vi "Assemble module.vi"() -> ()   [LabVIEW 2016]
uses:
  Classes/Assembly/Assembly Run.lvclass
  Classes/Routine/Routine Enum.ctl
  Classes/Workspace/Fixture Enum.ctl
  Classes/Routine/Routine.lvclass
  Classes/Workspace/Fixture.lvclass
  Classes/Controller/Controller.lvclass
panel:
  out "Routine Status":string
  in  "Add to Assembly":bool
  out "?":bool
  out "?":bool
  out "?":bool
  out "?":bool
  out "Theta":dbl
  out "Z":dbl
  out "Y":dbl
  out "X":dbl
  in  "Baseplate Tray ID":i32
  in  "Component Tray ID":i32
  out "Baseplate tray vacuum":bool
  out "Component Tray Vacuum":bool
  out "O-ring vacuum":bool
  out "Assembly vacuum":bool
  out "Component vacuum":bool
  out "Secondary vacuum":bool
  out "Primary vacuum":bool
  in  "Stop":bool
  in  "Number of modules":i32
  in  "Glue step":enum16{"Kapton", "Sensor", "PCB"}(ring)
  in  "Go":bool
  # "Status"
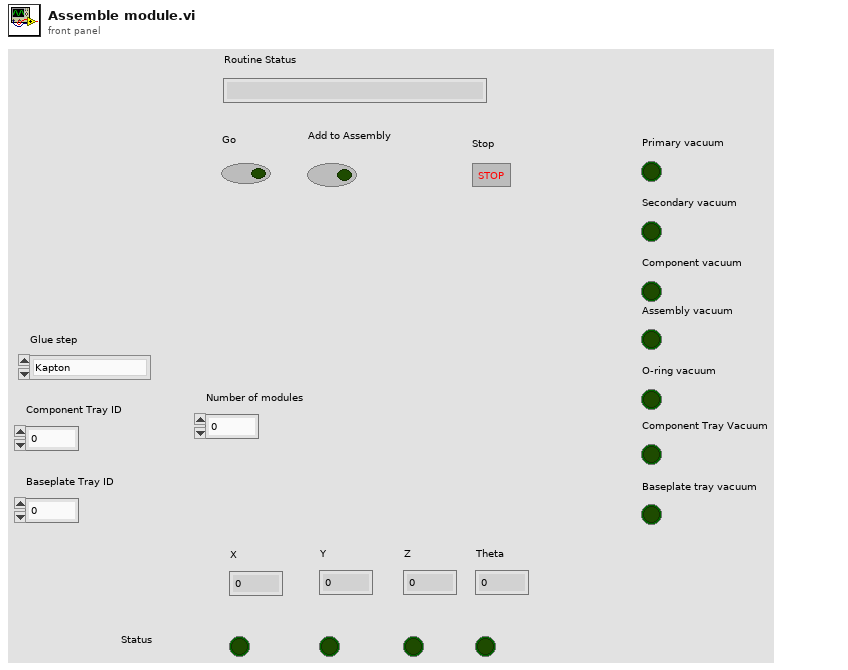
[diagram p1: front panel]
types:
  T1 = typedef "Fixture.lvclass/Fixture Enum.ctl" = enum16{"Assembly Tray", "Syringe Space", "Component", "Pick Up Tool", "Current Position"}
  T2 = typedef "Routine.lvclass/Routine Enum.ctl" = enum16{"Primary Pick Up", "Pick Up All", "Put Down Secondary", "Put Down All", "Release Syringe", "Secondary Pick Up", "Secure Syringe", "Dispense on Plate", "Dispense on Kapton", "Dispense on Sensor"}
  T3 = typedef "Controller.lvclass/Controllers.ctl" = cluster{"I-O.lvclass":refnum<class "I-O.lvclass">, "Motion.lvclass":refnum<class "Motion.lvclass">, "Dispenser.lvclass":refnum<class "Dispenser.lvclass">}
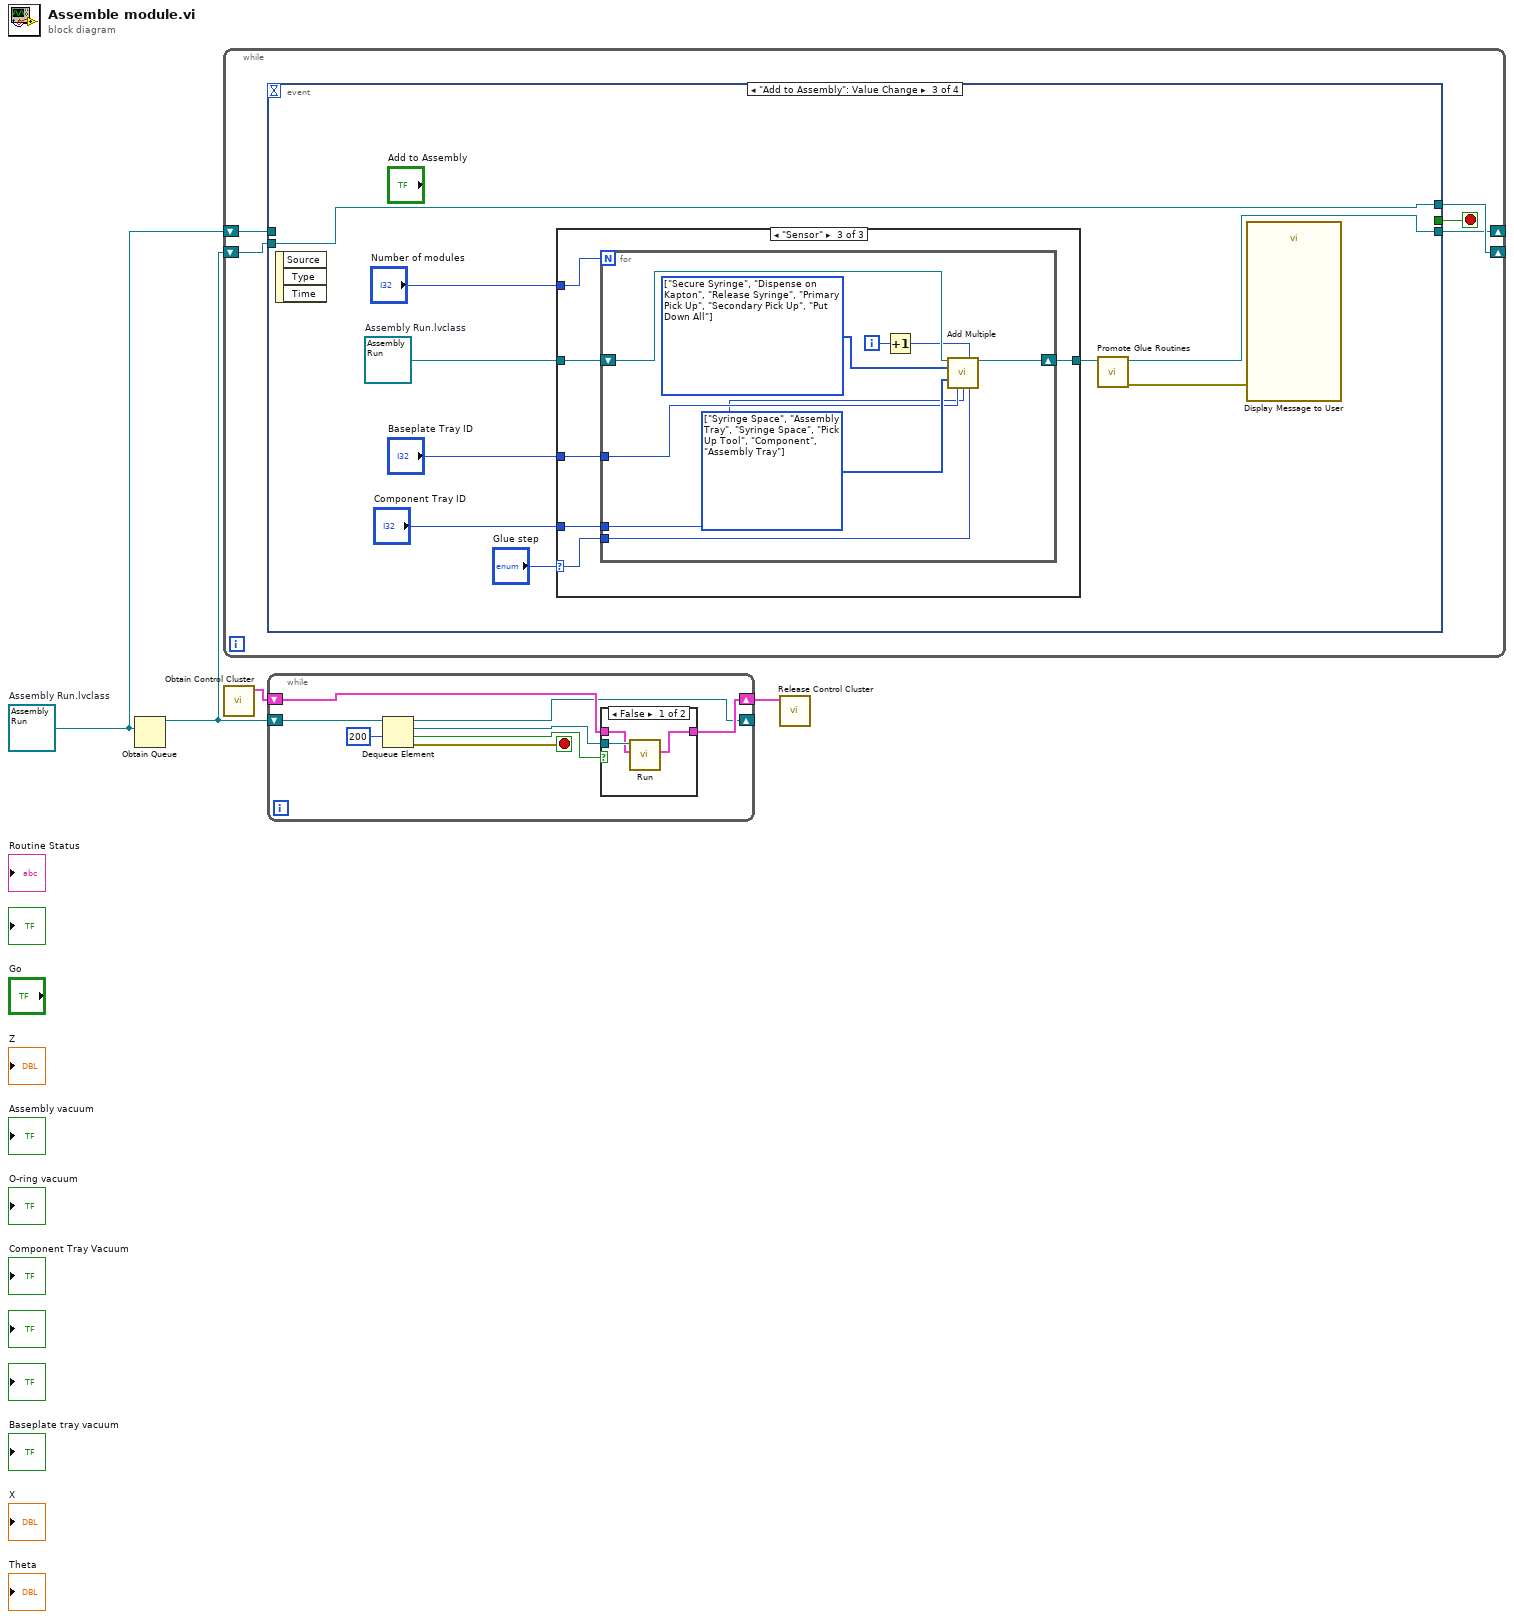
[diagram p0: block diagram]
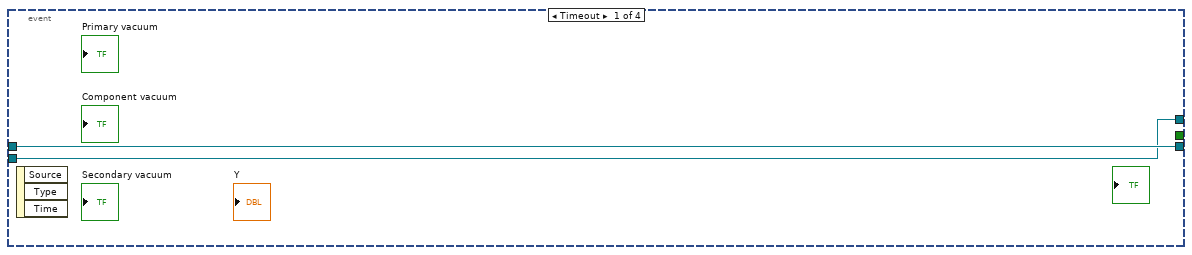
[diagram p3: hidden frame]
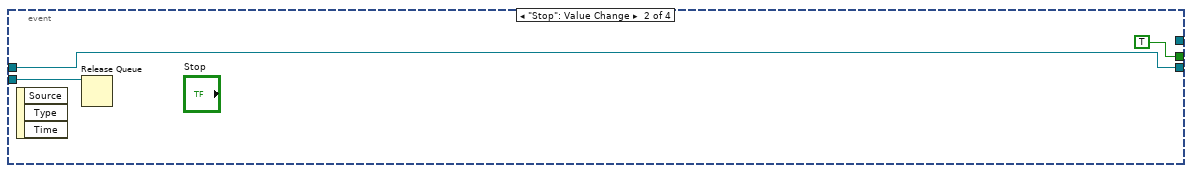
[diagram p4: hidden frame]
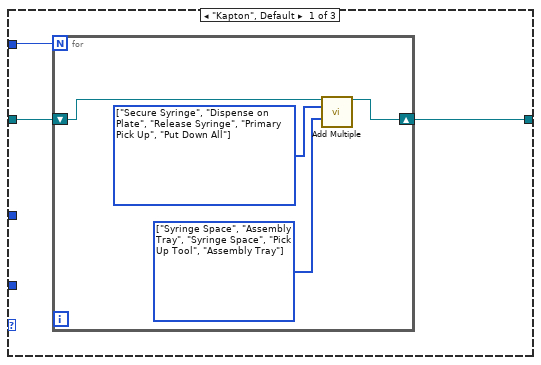
[diagram p5: hidden frame]
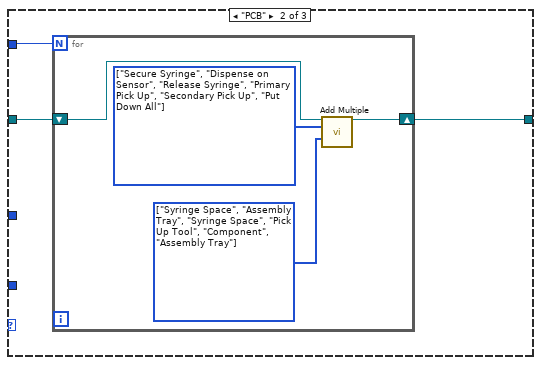
[diagram p6: hidden frame]
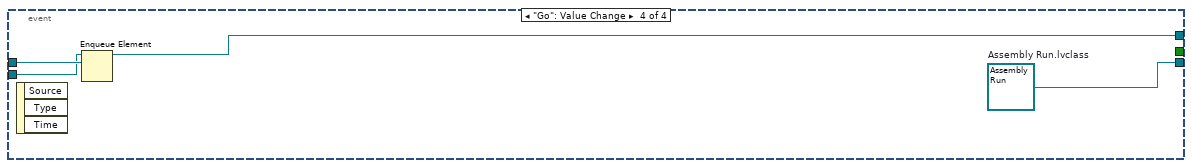
[diagram p7: hidden frame]
diagram:
  w2 = refnum<class "Assembly Run.lvclass"> refnum  # Assembly Run.lvclass
  n1 = Obtain Queue(element data type=w2) -> (queue out=w4:refnum<queue>)  [unwired: 4 in, 2 out]
  n2 = while {
    shift-right: [w8] -> _
    shift-left: w4 -> [w9]
    shift-right: [w6] -> _
    shift-left: w2 -> [w5]
    stop <- w7 stop-if-true
    n3 = event shown="[2] \"Add to Assembly\": Value Change" {
      selector: _ -> [_ _ _ _]
      dyn-events: _ -> [_ _ _ _]
      timeout: _ -> [_ _ _ _]
      tunnel: w9 -> [w10 w13 w21 w55]
      tunnel: [w10 _ w21 w54] -> w8
      tunnel: [_ TRUE _ _] -> w7
      tunnel: [w11 w12 w18 w53] -> w6
      tunnel: w5 -> [w11 w12 _ w56]
      event Timeout {
        n4 = event-data() -> ()  [unwired: 1 in, 3 out]
      }
      event "Stop": Value Change {
        n5 = event-data() -> ()  [unwired: 1 in, 3 out]
        n6 = Release Queue(queue=w13) -> ()  [unwired: 2 in, 3 out]
      }
      event "Add to Assembly": Value Change {
        w22 = refnum<class "Assembly Run.lvclass"> refnum  # Assembly Run.lvclass
        n7 = event-data() -> ()  [unwired: 1 in, 3 out]
        n8 = case shown="\"Sensor\"" "Glue step" {
          selector: "Glue step" -> [_ _ w38]
          tunnel: w22 -> [w25 w33 w39]
          tunnel: [w26 w32 w43] -> w19
          tunnel: "Number of modules" -> [w24 w31 w42]
          tunnel: "Component Tray ID" -> [_ _ w41]
          tunnel: "Baseplate Tray ID" -> [_ _ w40]
          frame "Kapton", Default {
            n9 = for {
              N: w24 -> [_]
              shift-right: [w29] -> w26
              shift-left: w25 -> [w30]
              w28 = T1[] [enum."Syringe Space", enum."Assembly Tray", enum."Syringe Space", enum."Pick Up Tool", enum."Assembly Tray"] items=["Assembly Tray", "Syringe Space", "Component", "Pick Up Tool", "Current Position"] ("Fixtures")
              w27 = T2[] [enum."Secure Syringe", enum."Dispense on Plate", enum."Release Syringe", enum."Primary Pick Up", enum."Put Down All"] items=["Primary Pick Up", "Pick Up All", "Put Down Secondary", "Put Down All", "Release Syringe", "Secondary Pick Up", "Secure Syringe", "Dispense on Plate", "Dispense on Kapton", "Dispense on Sensor"] ("Routine")
              n10 = call-dynamic "Add Multiple.vi"("Assembly in"=w30, "Routine"=w27, "Fixtures"=w28) -> ("Assembly out"=w29:refnum<class "Assembly Run.lvclass">)  [unwired: 11 in, 1 out]
            }
          }
          frame "PCB" {
            n11 = for {
              N: w31 -> [_]
              shift-right: [w36] -> w32
              shift-left: w33 -> [w37]
              w34 = T1[] [enum."Syringe Space", enum."Assembly Tray", enum."Syringe Space", enum."Pick Up Tool", enum."Component", enum."Assembly Tray"] items=["Assembly Tray", "Syringe Space", "Component", "Pick Up Tool", "Current Position"] ("Fixtures")
              w35 = T2[] [enum."Secure Syringe", enum."Dispense on Sensor", enum."Release Syringe", enum."Primary Pick Up", enum."Secondary Pick Up", enum."Put Down All"] items=["Primary Pick Up", "Pick Up All", "Put Down Secondary", "Put Down All", "Release Syringe", "Secondary Pick Up", "Secure Syringe", "Dispense on Plate", "Dispense on Kapton", "Dispense on Sensor"] ("Routine")
              n12 = call-dynamic "Add Multiple.vi"("Assembly in"=w37, "Routine"=w35, "Fixtures"=w34) -> ("Assembly out"=w36:refnum<class "Assembly Run.lvclass">)  [unwired: 11 in, 1 out]
            }
          }
          frame "Sensor" {
            n13 = for {
              N: w42 -> [_]
              shift-right: [w51] -> w43
              shift-left: w39 -> [w52]
              tunnel: w41 -> [w47]
              tunnel: w40 -> [w48]
              tunnel: w38 -> [w44]
              i -> [w46]
              w49 = T1[] [enum."Syringe Space", enum."Assembly Tray", enum."Syringe Space", enum."Pick Up Tool", enum."Component", enum."Assembly Tray"] items=["Assembly Tray", "Syringe Space", "Component", "Pick Up Tool", "Current Position"] ("Fixtures")
              w50 = T2[] [enum."Secure Syringe", enum."Dispense on Kapton", enum."Release Syringe", enum."Primary Pick Up", enum."Secondary Pick Up", enum."Put Down All"] items=["Primary Pick Up", "Pick Up All", "Put Down Secondary", "Put Down All", "Release Syringe", "Secondary Pick Up", "Secure Syringe", "Dispense on Plate", "Dispense on Kapton", "Dispense on Sensor"] ("Routine")
              n14 = Increment(x=w46) -> (x+1=w45:i32)
              n15 = call-dynamic "Add Multiple.vi"("Assembly in"=w52, "Position"=w45, "Routine"=w50, "Fixtures"=w49, "Baseplate Tray ID"=w48, "Component Tray ID"=w47, "Glue step"=w44) -> ("Assembly out"=w51:refnum<class "Assembly Run.lvclass">)  [unwired: 7 in, 1 out]
            }
          }
        }
        n16 = call "Promote Glue Routines.vi"("Assembly Run in"=w19) -> ("error out"=w15:errorcluster, "Assembly Run out"=w18:refnum<class "Assembly Run.lvclass">)  [unwired: 9 in]
        n17 = call "Display Message to User"("error in (no error)"=w15) -> ()  [unwired: 9 in, 2 out]
      }
      event "Go": Value Change {
        w53 = refnum<class "Assembly Run.lvclass"> refnum  # Assembly Run.lvclass
        n18 = event-data() -> ()  [unwired: 1 in, 3 out]
        n19 = Enqueue Element(queue=w55, element=w56) -> (queue out=w54:refnum<queue>)  [unwired: 2 in, 2 out]
      }
    }
  }
  n20 = call "Obtain Control Cluster.vi"() -> ("Control Out"=w3:T3)  [unwired: 11 in]
  n21 = while {
    shift-right: [w57] -> _
    shift-left: w4 -> [w64]
    shift-right: [w59] -> w1
    shift-left: w3 -> [w60]
    stop <- w58 stop-if-true
    n22 = Dequeue Element(queue=w64, timeout in ms (-1)=200) -> (queue out=w57:refnum<queue>, element=w63:refnum<class "Assembly Run.lvclass">, timed out?=w62:bool, error out=w58:errorcluster)  [unwired: 1 in]
    n23 = case shown="False" w62 {
      tunnel: w63 -> [w67 _]
      tunnel: w60 -> [w66 w68]
      tunnel: [w65 w68] -> w59
      frame False {
        n24 = call-dynamic "Run.vi"("Control In"=w66, "Assembly In"=w67) -> ("Control Out"=w65:T3)  [unwired: 7 in, 2 out]
      }
      frame True {
      }
    }
  }
  n25 = call "Release Control Cluster.vi"("output cluster"=w1) -> ()  [unwired: 11 in]
